vi "ClarkeFXP_src.vi"(0 "A":fxp<+/-,32,4>, 5 "B":fxp<+/-,32,4>, 7 "C":fxp<+/-,32,4>) -> (4 "alpha":fxp<+/-,32,4>, 6 "beta":fxp<+/-,32,4>)   [LabVIEW 2016]
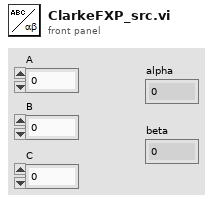
[diagram p1: front panel]
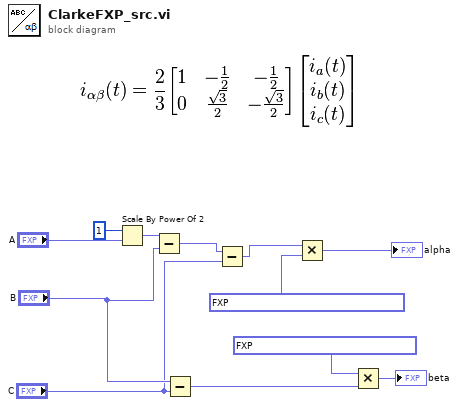
[diagram p0: block diagram]
diagram:
  n1 = Scale By Power Of 2(n=i16 1, x="A") -> (x*2^n=w6:fxp<+/-,32,4>)
  n2 = Subtract(x=w6, y="B") -> (x-y=w4:fxp<+/-,33,5>)
  n3 = Subtract(x="B", y="C") -> (x-y=w3:fxp<+/-,33,5>)
  n4 = Subtract(x=w4, y="C") -> (x-y=w2:fxp<+/-,34,6>)
  n5 = Multiply(x=w2, y=fxp<+,31,-1> 0.3333333330228925) -> (x*y=→"alpha":fxp<+/-,64,4>)
  n6 = Multiply(x=fxp<+/-,32,4> 0.5773500017821789, y=w3) -> (x*y=→"beta":fxp<+/-,64,8>)
